vi "Jacobian.vi"() -> ()   [LabVIEW 2020, in "Examples.lvlib"]
uses:
  Examples.lvlib
  classes/Dual/Dual.lvclass/Dual.ctl
  Automatic Differentiation/Evaluate Jacobian.vi/d3fc5611-aad1-4343-aaaf-f0a6943ff05c.vi
  classes/Dual/Add infinitesimal to Double.vi
  classes/Dual/Read Dual Part.vi
  Automatic Differentiation/Evaluate Jacobian.vi/d3fc5611-aad1-4343-aaaf-f0a6943ff05c.vi/5957e011-cf56-4527-b6ed-13c3a4ca997b.vi
  classes/Dual/Write a.vi
  Tests/Vector-valued Function.vi
  classes/Dual/Dual.lvclass
  Automatic Differentiation/Automatic Differentiation.lvlib
  Tests/Tests.lvlib
panel:
  out "Df(x)":dbl[][](array[numeric])
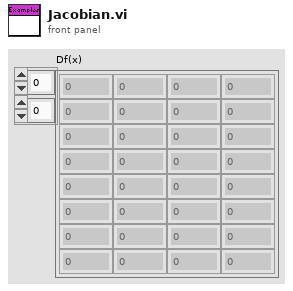
[diagram p1: front panel]
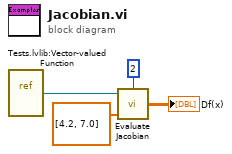
[diagram p0: block diagram]
diagram:
  n1 = vi-ref "Tests.lvlib:Vector-valued Function.vi"() -> (w4:refnum<vi>)
  n2 = call "Evaluate Jacobian.vi"("m"=2, "Point (x_1, ..., x_n)"=dbl[] [4.2, 7.0] ("Point (x_1,...,x_n)"), "Function Reference"=w4) -> ("Df(x)"=→"Df(x)":dbl[][])  [unwired: 1 in]
